vi "MT Calculate Scaling Factor (ASK).vi"(5 "ASK system parameters":T1 {"symbol map" format="%.3f"}, 7 "pulse shaping filter coefficients":dbl[](array[numeric]) format="%.2f", 11 "error in (no error)":errorcluster) -> (6 "waveform scaling factor":dbl, 15 "error out":errorcluster)   [LabVIEW 2020, in "niDMT.lvlib"]
doc: "Calculates the maximum possible waveform amplitude for the ASK modulation scheme."
uses:
  <vilib>/addons/Modulation/niDMT.lvlib
  <vilib>/addons/Modulation/Digital/Support/Common/Validators/mod_Validate Symbol Map (PAM).vi
  <vilib>/addons/Modulation/Digital/Support/Common/Validators/mod_Validate Symbol Map Collinearity.vi
  <vilib>/Analysis/6fits.llb/Linear Fit.vi
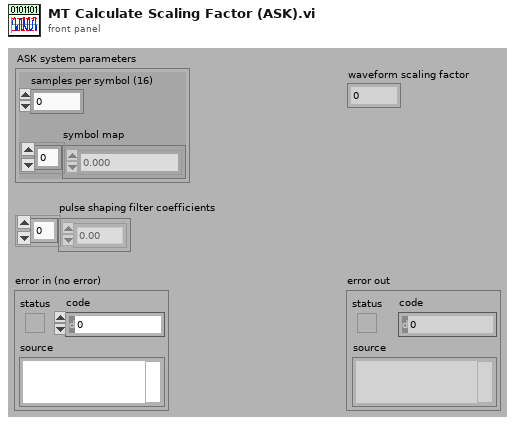
[diagram p1: front panel]
types:
  T1 = cluster{"samples per symbol (16)":i32, "symbol map":cdb[]}
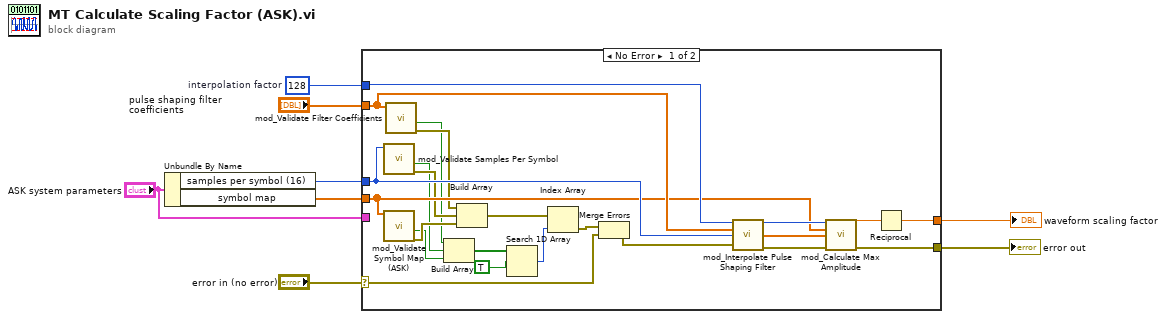
[diagram p0: block diagram]
diagram:
  w8 = 128  # interpolation factor
  n1 = Unbundle By Name("ASK system parameters") -> ("samples per symbol (16)"=w3:i32, "symbol map"=w2:cdb[])
  n2 = case shown="No Error" "error in (no error)" {
    selector: "error in (no error)" -> [w9 w32]
    tunnel: w8 -> [w31 _]
    tunnel: [w27 _] -> w7
    tunnel: "pulse shaping filter coefficients" -> [w26 _]
    tunnel: w3 -> [w25 _]
    tunnel: [w21 w32] -> w4
    tunnel: w2 -> [w24 _]
    tunnel: "ASK system parameters" -> [_ _]
    frame No Error {
      n3 = call <vilib>:"mod_Validate Samples Per Symbol.vi"("Samples Per Symbol"=w25) -> ("error out"=w19:errorcluster, "error?"=w16:bool)  [unwired: 9 out]
      n4 = call <vilib>:"mod_Validate Symbol Map (ASK).vi"("Symbol Map"=w24) -> ("error out"=w18:errorcluster, "error?"=w15:bool)  [unwired: 9 out]
      n5 = call <vilib>:"mod_Validate Filter Coefficients.vi"("Filter Coefficients"=w26) -> ("error out"=w20:errorcluster, "error?"=w17:bool)  [unwired: 9 out]
      n6 = Build Array(w17, w16, w15) -> (w14:bool[])
      n7 = Build Array(w20, w19, w18) -> (w12:errorcluster[])
      n8 = Search 1D Array(1D array=w14, element=TRUE) -> (index of element=w11:i32)  [unwired: 1 out]
      n9 = Index Array(array=w12, index=w11) -> (element=w10:errorcluster)
      n10 = Merge Errors(w10, w9) -> (w22:errorcluster)
      n11 = call <vilib>:"mod_Interpolate Pulse Shaping Filter.vi"("interpolation factor"=w31, "pulse shaping filter coefficients in"=w26, "samples per symbol  in (16 )"=w25, "error in (no error)"=w22) -> ("samples per symbol out (16)"=w29:i32, "pulse shaping filter coefficients out"=w30:dbl[], "error out"=w23:errorcluster)  [unwired: 9 out]
      n12 = call <vilib>:"mod_Calculate Max Amplitude.vi"("pulse shaping samples per symbol (16)"=w29, "symbol map"=w24, "pulse shaping filter coefficients"=w30, "error in (no error)"=w23) -> ("Max. Amplitude (worst case)"=w28:dbl, "error out"=w21:errorcluster)  [unwired: 10 out]
      n13 = Reciprocal(x=w28) -> (1/x=w27:dbl)
    }
    frame Error {
    }
  }
  "waveform scaling factor" <- w7
  "error out" <- w4
